vi "ClimbTeleop.vi"(7 "ClimbCancel":bool, 8 "ClimbPull":bool, 9 "ClimbReach":bool, 10 "ClimbIncPull":bool, 11 "ClimbIncReach":bool) -> ()   [LabVIEW 2023]
doc: "Sends various SendCmds if corresponding inputs are \"true\""
uses:
  <vilib>/Rock Robotics/WPI/ThirdParty/JAS_Junk/TrajLib/VI/BoolCmd_Send.vi
  <vilib>/Rock Robotics/WPI/ThirdParty/JAS_Junk/TrajLib/VI/BoolCmd_Send_Internal.vi
  <vilib>/Rock Robotics/WPI/ThirdParty/JAS_Junk/TrajLib/VI/BoolCmd_ObtainQueue.vi
  <vilib>/Rock Robotics/WPI/ThirdParty/JAS_Junk/TrajLib/Trajectory_Library.lvlib
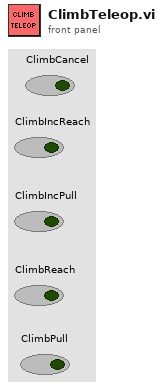
[diagram p1: front panel]
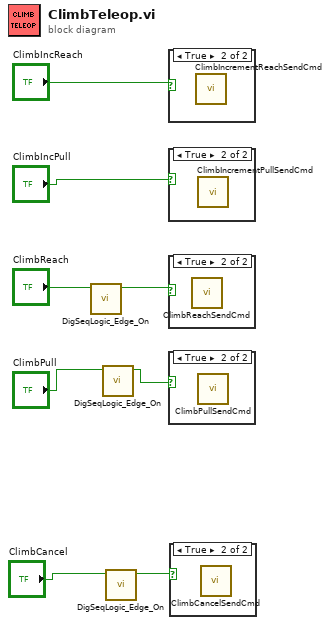
[diagram p0: block diagram]
diagram:
  n1 = call <vilib>:"DigSeqLogic_Edge_On.vi"("Input"="ClimbReach") -> ("On Edge"=w5:bool)  [unwired: 10 in]
  n2 = call <vilib>:"DigSeqLogic_Edge_On.vi"("Input"="ClimbPull") -> ("On Edge"=w1:bool)  [unwired: 10 in]
  n3 = call <vilib>:"DigSeqLogic_Edge_On.vi"("Input"="ClimbCancel") -> ("On Edge"=w3:bool)  [unwired: 10 in]
  n4 = case shown="True" "ClimbIncReach" {
    frame False {
    }
    frame True {
      n5 = call "ClimbIncrementReachSendCmd.vi"() -> ()  [unwired: 12 in]
    }
  }
  n6 = case shown="True" "ClimbIncPull" {
    frame False {
    }
    frame True {
      n7 = call "ClimbIncrementPullSendCmd.vi"() -> ()  [unwired: 12 in]
    }
  }
  n8 = case shown="True" w5 {
    frame False {
    }
    frame True {
      n9 = call "ClimbReachSendCmd.vi"() -> ()  [unwired: 12 in]
    }
  }
  n10 = case shown="True" w1 {
    frame False {
    }
    frame True {
      n11 = call "ClimbPullSendCmd.vi"() -> ()  [unwired: 12 in]
    }
  }
  n12 = case shown="True" w3 {
    frame False {
    }
    frame True {
      n13 = call "ClimbCancelSendCmd.vi"() -> ()  [unwired: 12 in]
    }
  }
